vi "ClusterToArray.vi"(3 "State_n_n":T1) -> (0 "State Array":dbl[](array[numeric]), 1 "N_r":i32, 2 "N_c":i32)   [LabVIEW 2019]
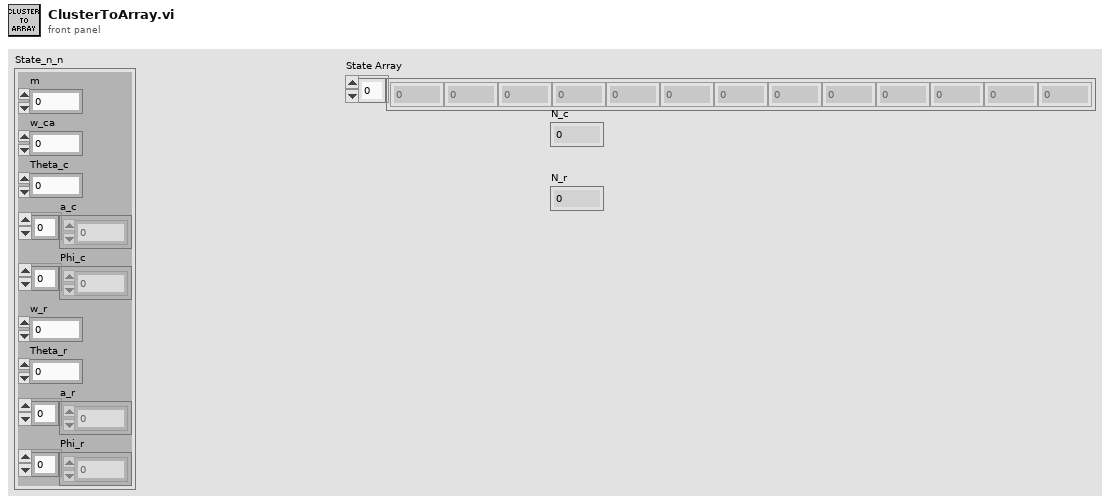
[diagram p1: front panel]
types:
  T1 = cluster{"m":dbl, "w_ca":dbl, "Theta_c":dbl, "a_c":dbl[], "Phi_c":dbl[], "w_r":dbl, "Theta_r":dbl, "a_r":dbl[], "Phi_r":dbl[]}
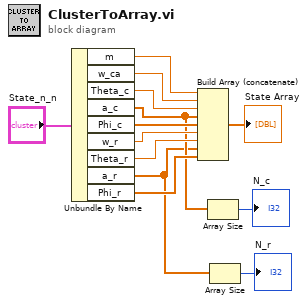
[diagram p0: block diagram]
diagram:
  n1 = Unbundle By Name("State_n_n") -> ("m"=w11:dbl, "w_ca"=w10:dbl, "Theta_c"=w9:dbl, "a_c"=w4:dbl[], "Phi_c"=w8:dbl[], "w_r"=w7:dbl, "Theta_r"=w6:dbl, "a_r"=w1:dbl[], "Phi_r"=w5:dbl[])
  n2 = Build Array (concatenate)(w11, w10, w9, w4, w8, w7, w6, w1, w5) -> (→"State Array":dbl[])
  n3 = Array Size(array=w4) -> (size(s)=→"N_c":i32)
  n4 = Array Size(array=w1) -> (size(s)=→"N_r":i32)
